vi "Close Session.vi"(8 "error in (no error)":errorcluster, 11 "Session in":refnum<class "Plugin Session.lvclass">) -> (0 "error out":errorcluster)   [LabVIEW 2021, in "InstrumentStudio Plugin SDK.lvlib" / "Plugin Session.lvclass"]
doc: "Call this VI to close out all references created for the session and unregister the plugin session with the framework. It should be called at the end of your plugin VI after the event loop is completed as the last call in the VI."
uses:
  Plugin Session.lvclass
  Plugin Session.lvclass/Plugin Session.ctl
  Plugin Events.ctl
  Event Registration Refnum.ctl
  Read Plugin Events.vi
  Read Event Refnum.vi
  InstrumentStudio Plugin SDK.lvlib
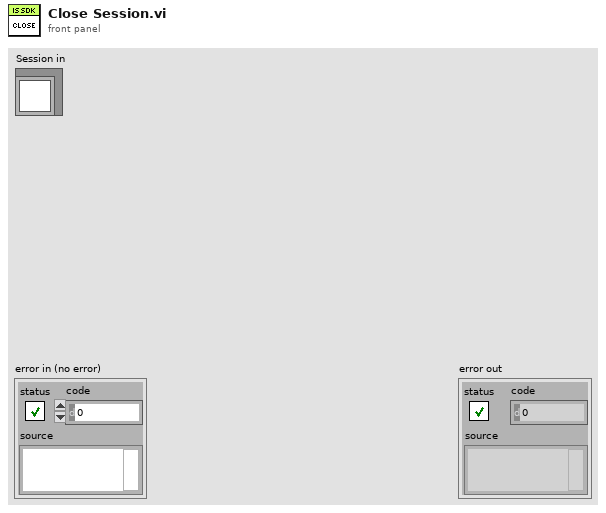
[diagram p1: front panel]
types:
  T1 = typedef "InstrumentStudio Plugin SDK.lvlib/Plugin Events.ctl" = cluster{"Shutdown":refnum<user-event>, "Project Saved":refnum<user-event>, "Stop All Outputs":refnum<user-event>, "Generic Message":refnum<user-event>}
  T2 = typedef "InstrumentStudio Plugin SDK.lvlib/Event Registration Refnum.ctl" = refnum<event-registration>
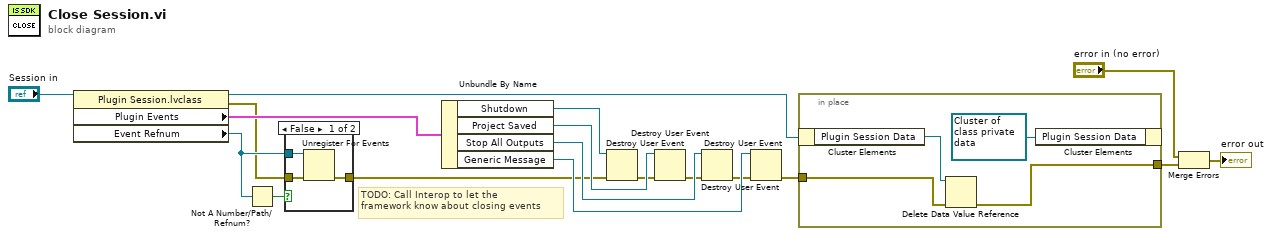
[diagram p0: block diagram]
diagram:
  # "TODO: Call Interop to let the\nframework know about closing events"
  n1 = property class="Plugin Session.lvclass"(reference="Session in") -> (reference out=w6:refnum<class "Plugin Session.lvclass">, error out=w5:errorcluster, "Plugin Events"=w14:T1, "Event Refnum"=w11:T2)  [unwired: 1 in]
  n2 = Not A Number/Path/Refnum?(number/path/refnum=w11) -> (NaN/Path/Refnum?=w15:bool)
  n3 = case shown="False" w15 {
    tunnel: [w21 w22] -> w10
    tunnel: w11 -> [w20 _]
    tunnel: w5 -> [w19 w22]
    frame False {
      n4 = Unregister For Events(event registration refnum=w20, error in=w19) -> (error out=w21:errorcluster)
    }
    frame True {
    }
  }
  n5 = Unbundle By Name(w14) -> ("Shutdown"=w13:refnum<user-event>, "Project Saved"=w12:refnum<user-event>, "Stop All Outputs"=w17:refnum<user-event>, "Generic Message"=w18:refnum<user-event>)
  n6 = Destroy User Event(user event=w13, error in=w10) -> (error out=w1:errorcluster)
  n7 = Destroy User Event(user event=w12, error in=w1) -> (error out=w4:errorcluster)
  n8 = Destroy User Event(user event=w17, error in=w4) -> (error out=w3:errorcluster)
  n9 = Destroy User Event(user event=w18, error in=w3) -> (error out=w2:errorcluster)
  n10 = in-place {
    in-place-border: w2 -> [w26]
    in-place-border: [w24] -> w7
    n11 = in-place-cluster #1(w6) -> ("Plugin Session Data"=w25:refnum<data-value>)
    n12 = Delete Data Value Reference(data value reference=w25, error in=w26) -> (error out=w24:errorcluster)  [unwired: 1 out]
    n13 = in-place-cluster #1("Plugin Session Data"=refnum<data-value> refnum) -> ()  [unwired: 1 out]
  }
  n14 = Merge Errors("error in (no error)", w7) -> (→"error out":errorcluster)
